vi "Configure TILT Unit.vi"(8 "error in (no error)":errorcluster, 10 "Unit (1: DB)":i32(ring)=1 items=["PCT", "DB"], 11 "VISA resource name":refnum<visa-resource-name>) -> (0 "error out":errorcluster, 3 "VISA resource name out":refnum<visa-resource-name>)   [LabVIEW 2014, in "Agilent U2000 Series.lvlib"]
doc: "Sets the unit for the tilt (droop) measurement.\n\nNote: \nThis VI is only applicable for U2042XA/U2044XA/U2049XA."
uses:
  Agilent U2000 Series.lvlib
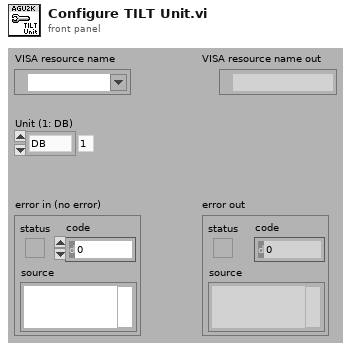
[diagram p1: front panel]
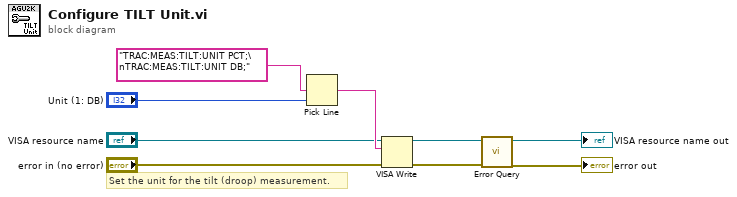
[diagram p0: block diagram]
diagram:
  # "Set the unit for the tilt (droop) measurement."
  n1 = Pick Line(multi-line string="TRAC:MEAS:TILT:UNIT PCT;\nTRAC:MEAS:TILT:UNIT DB;", line index="Unit (1: DB)") -> (output string=w7:string)  [unwired: 1 in]
  n2 = VISA Write(VISA resource name="VISA resource name", write buffer=w7, error in (no error)="error in (no error)") -> (VISA resource name out=w4:refnum<visa-resource-name>, error out=w3:errorcluster)  [unwired: 1 out]
  n3 = call "Error Query.vi"("error in (no error)"=w3, "VISA resource name"=w4) -> ("error out"=→"error out":errorcluster, "VISA resource name out"=→"VISA resource name out":refnum<visa-resource-name>)  [unwired: 6 in, 2 out]
